vi "DSF.Shared.Configuration.Framework.Get Unique Name.Transfer.vi"(8 "error in (no error)":errorcluster, 11 "Framework Configuration in":refnum<class "DSF.Shared.Configuration.Framework.lvclass">) -> (0 "error out":errorcluster, 2 "unique name":string, 3 "Framework Configuration out":refnum<class "DSF.Shared.Configuration.Framework.lvclass">)   [LabVIEW 2017, in "DSF.Shared.lvlib" / "DSF.Shared.Configuration.Framework.lvclass"]
uses:
  DSF.Shared.Configuration.Framework.lvclass
  DSF.Shared.Configuration.Framework.lvclass/DSF.Shared.Configuration.Framework.ctl
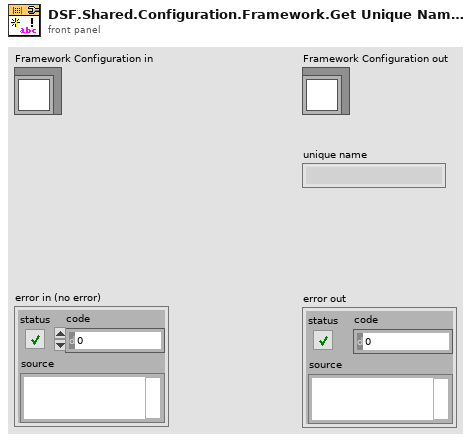
[diagram p1: front panel]
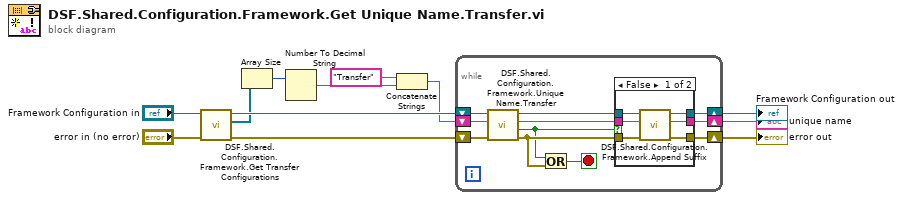
[diagram p0: block diagram]
diagram:
  n1 = call "DSF.Shared.Configuration.Framework.Get Transfer Configurations.vi"("Framework Configuration in"="Framework Configuration in") -> ("Transfer Configurations"=w3:refnum<class "DSF.Shared.Configuration.Transfer.lvclass">[], "Framework Configuration out"=w4:refnum<class "DSF.Shared.Configuration.Framework.lvclass">)  [unwired: 9 in]
  n2 = Array Size(array=w3) -> (size(s)=w7:i32)
  n3 = Number To Decimal String(number=w7) -> (decimal integer string=w6:string)  [unwired: 1 in]
  n4 = Concatenate Strings("Transfer" ("name"), w6) -> (w2:string)
  n5 = while {
    shift-right: [w19] -> w9
    shift-left: w4 -> [w20]
    shift-right: [w17] -> w11
    shift-left: "error in (no error)" -> [w18]
    shift-right: [w15] -> w1
    shift-left: w2 -> [w21]
    stop <- w12 stop-if-true
    n6 = call "DSF.Shared.Configuration.Framework.Unique Name.Transfer.vi"("error in (no error)"=w18, "Transfer name in"=w21, "Framework Configuration in"=w20) -> ("error out"=w14:errorcluster, "unique Transfer name?"=w13:bool, "Transfer name out"=w16:string, "Framework Configuration out"=w22:refnum<class "DSF.Shared.Configuration.Framework.lvclass">)  [unwired: 5 in]
    n7 = Or(x=w13, y=w14) -> (x .or. y?=w12:bool)
    n8 = case shown="False" w13 {
      tunnel: w22 -> [w28 w31]
      tunnel: w14 -> [w27 w30]
      tunnel: w16 -> [w26 w29]
      tunnel: [w25 w29] -> w15
      tunnel: [w24 w30] -> w17
      tunnel: [w23 w31] -> w19
      frame False {
        n9 = call "DSF.Shared.Configuration.Framework.Append Suffix.vi"("error in (no error)"=w27, "string"=w26, "Framework Configuration in"=w28) -> ("error out"=w24:errorcluster, "appended string"=w25:string, "Framework Configuration out"=w23:refnum<class "DSF.Shared.Configuration.Framework.lvclass">)  [unwired: 6 in]
      }
      frame True {
      }
    }
  }
  "error out" <- w11
  "Framework Configuration out" <- w9
  "unique name" <- w1
